vi "Begin.vi"(8 "error in":errorcluster) -> (0 "error out":errorcluster)   [LabVIEW 2019]
doc: "Called before other user functions, this VI is expected to open initial I/O refnums, load in file data, and do all program initialization. Notice that the <B>error out</B> terminal is simply used for data flow. Wiring it to other structures or subVIs ensures that this VI runs first."
uses:
  <vilib>/Rock Robotics/WPI/DriverStation/WPI_DriverStationRobotMode2.ctl
  <vilib>/Rock Robotics/WPI/Joystick/WPI_JoystickDeviceEnum.ctl
  <vilib>/Rock Robotics/SystemInterfaces/i2clib/i2c_bus.ctl
  <vilib>/Rock Robotics/WPI/ThirdParty/REV Robotics/Color SensorV3/Typedef/Color Sensor V3 LEDPulseFreq.ctl
  <vilib>/Rock Robotics/WPI/ThirdParty/REV Robotics/Color SensorV3/Typedef/Color Sensor V3 LEDCurrent.ctl
  <vilib>/Rock Robotics/SystemInterfaces/DIO/FPGA_DIOPWMChannel.ctl
  <vilib>/Rock Robotics/WPI/SafetyOutput/WPI_SafetyOutputConfigMenu.ctl
  <vilib>/Rock Robotics/SystemInterfaces/AI/FPGA_AIChannel.ctl
  <vilib>/Rock Robotics/WPI/Solenoid/WPI_SolenoidChannel.ctl
  Robot Global Data.vi
  <vilib>/Rock Robotics/Network Tables/NT Write String Array.vi
  Downloads/Global 2.vi
  <vilib>/Rock Robotics/WPI/Ultrasonic/WPI_SonarMB1010AnalogOpen.vi
  <vilib>/Rock Robotics/WPI/Ultrasonic/WPI_SonarMB1010AnalogRefNum Registry Set.vi
  <vilib>/Rock Robotics/WPI/MotorControl/WPI_MotorControlOpen VictorSPX.vi
  <vilib>/Rock Robotics/WPI/MotorControl/WPI_MotorControlOpen Talon.vi
  <vilib>/Rock Robotics/WPI/Solenoid/WPI_SolenoidOpenSingle.vi
  <vilib>/Rock Robotics/WPI/RobotDrive/WPI_RobotDriveOpen4MotorWithSPARK.vi
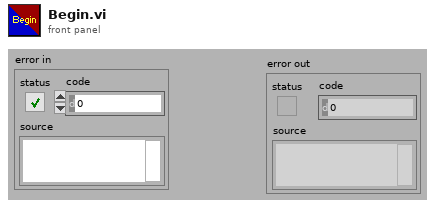
[diagram p1: front panel]
types:
  T1 = typedef "WPI_SolenoidChannel.ctl" = enum8{"Solenoid 0", "Solenoid 1", "Solenoid 2", "Solenoid 3", "Solenoid 4", "Solenoid 5", "Solenoid 6", "Solenoid 7", "Invalid"}
  T2 = typedef "FPGA_DIOPWMChannel.ctl" = enum8{"PWM 0", "PWM 1", "PWM 2", "PWM 3", "PWM 4", "PWM 5", "PWM 6", "PWM 7", "PWM 8", "PWM 9", "PWM MXP 0", "PWM MXP 1", "PWM MXP 2", "PWM MXP 3", "PWM MXP 4", "PWM MXP 5", "PWM MXP 6", "PWM MXP 7", "PWM MXP 8", "PWM MXP 9", "Invalid"}
  T3 = typedef "FPGA_AIChannel.ctl" = enum8{"AI 0", "AI 1", "AI 2", "AI 3", "AI MXP 0", "AI MXP 1", "AI MXP 2", "AI MXP 3", "Invalid"}
  T4 = typedef "WPI_SafetyOutputConfigMenu.ctl" = enum16{"Enable", "Disable"}
  T5 = typedef "Color Sensor V3 LEDCurrent.ctl" = enum8{"2.5mA", "5.0mA", "10mA", "25mA", "50mA", "75mA", "100mA", "125mA"}
  T6 = typedef "Color Sensor V3 LEDPulseFreq.ctl" = enum16{"60kHz", "70kHz", "80kHz", "90kHz", "100kHz"}
  T7 = typedef "i2c_bus.ctl" = enum16{"I2C On-Board", "I2C MXP", "Invalid"}
  T8 = typedef "WPI_JoystickDeviceEnum.ctl" = enum16{"USB 0", "USB 1", "USB 2", "USB 3", "USB 4", "USB 5"}
  T9 = typedef "WPI_DriverStationRobotMode2.ctl" = enum16{"Autonomous Disabled", "Autonomous Enabled", "Teleop Disabled", "Teleop Enabled", "Disconnected", "Finish", "Test Disabled", "Test Enabled", "Emergency Stopped"}
  T10 = typedef "WPI_RobotDriveDevRef.ctl" = cluster{"DevStatus":errorcluster, "Motors[]":T11[], "Square Inputs":bool, "Max Output":dbl}
  T11 = typedef "WPI_MotorControlDeviceRef.ctl" = cluster{"DeviceStatus":errorcluster, "Type":T12, "PWM":cluster{"PWM Channel":T2, "DeadBand":T13}, "CAN":cluster{"Device Number":u8, "SetOutput VI Ref":variant, "GetOutput VI Ref":variant, "Enable VI Ref":variant, "Disable VI Ref":variant, "Data":variant}, "Invert":bool, "DIO PWM":cluster{"PWM \"Enable\" Channel":T2, "DIOChannel":T14, "PWM Rate":dbl}}
  T12 = typedef "WPI_MotorControlType.ctl" = enum16{"PWM", "CAN", "DIO PWM"}
  T13 = typedef "WPI_PWMDeadband.ctl" = cluster{"Name":string, "maxPositivePwm":i32, "minPositivePwm":i32, "centerPwm":i32, "maxNegativePwm":i32, "minNegativePwm":i32, "angularRange":u16}
  T14 = typedef "FPGA_DIOChannel.ctl" = enum8{"DIO 0", "DIO 1", "DIO 2", "DIO 3", "DIO 4", "DIO 5", "DIO 6", "DIO 7", "DIO 8", "DIO 9", "DIO MXP 0", "DIO MXP 1", "DIO MXP 2", "DIO MXP 3", "DIO MXP 4", "DIO MXP 5", "DIO MXP 6", "DIO MXP 7", "DIO MXP 8", "DIO MXP 9", "DIO MXP 10", "DIO MXP 11", "DIO MXP 12", "DIO MXP 13", "DIO MXP 14", "DIO MXP 15", "SPI Port CS1", "SPI Port CS2", "SPI Port CS3", "SPI Port MISO", "SPI Port MOSI", "Invalid"}
  T15 = typedef "WPI_JoystickDevRef.ctl" = cluster{"Device":T8}
  T16 = typedef "Color Sensor V3 DevRef.ctl" = cluster{"I2CDevRef":T17}
  T17 = typedef "WPI_I2CDevRef.ctl" = cluster{"DevStatus":errorcluster, "Device Address":u8, "Handle":i32, "I2C Bus":T7}
  T18 = typedef "WPI_SolenoidDevRef.ctl" = cluster{"DevStatus":errorcluster, "Pneumatics Control Module":u8, "Forward Solenoid Channel":T1, "Reverse Solenoid Channel":T1}
  T19 = typedef "WPI_SonarMB1010AnalogDeviceRef.ctl" = cluster{"AIDeviceRef":T20, "Scaling factor (V/in)":dbl, "Average Bits":u8}
  T20 = typedef "WPI_AnalogChannelDevRef.ctl" = cluster{"DevStatus":errorcluster, "Analog Channel":T3}
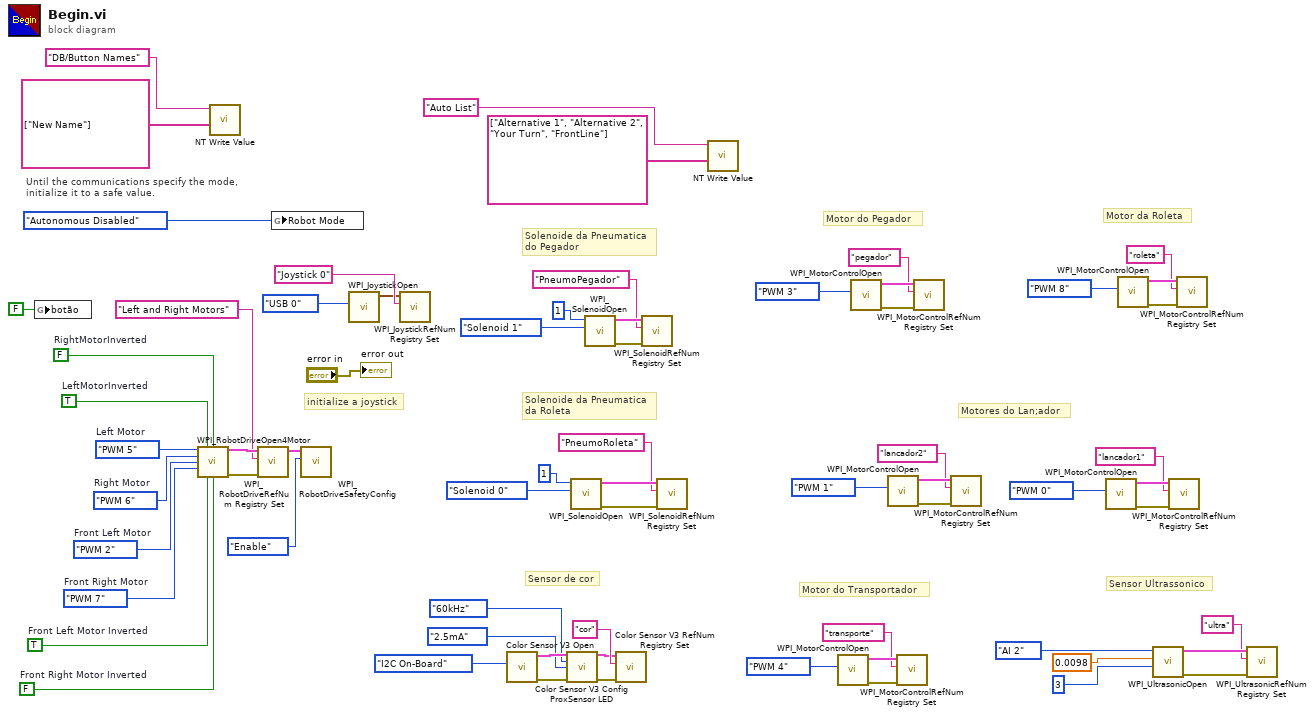
[diagram p0: block diagram]
diagram:
  w6 = FPGA_DIOPWMChannel."PWM 7"  # Front Right Motor
  w7 = FPGA_DIOPWMChannel."PWM 2"  # Front Left Motor
  w8 = FALSE  # Front Right Motor Inverted
  w9 = TRUE  # Front Left Motor Inverted
  w43 = FPGA_DIOPWMChannel."PWM 6"  # Right Motor
  w44 = FPGA_DIOPWMChannel."PWM 5"  # Left Motor
  w48 = TRUE  # LeftMotorInverted
  w49 = FALSE  # RightMotorInverted
  # "Sensor Ultrassonico"
  # "Motor do Transportador"
  # "Sensor de cor"
  # "Motores do Lan;ador"
  # "Motor da Roleta"
  # "Motor do Pegador"
  # "Solenoide da Pneumatica\nda Roleta"
  # "Solenoide da Pneumatica\ndo Pegador"
  # "initialize a joystick"
  # "Until the communications specify the mode,\ninitialize it to a safe value."
  n1 = global write "Global 2.vi" "botão"(FALSE ("botão")) -> ()
  n2 = call-poly <vilib>:"WPI_RobotDriveOpen4Motor.vi"("Rear Left Motor"=w44, "Rear Left Motor Inverted"=w48, "Rear Right Motor Inverted"=w49, "Rear Right Motor"=w43, "Front Left Motor"=w7, "Front Right Motor"=w6, "Front Left Motor Inverted"=w9, "Front Right Motor Inverted"=w8) -> ("RobotDriveDevRef"=w47:T10, "error out"=w45:errorcluster)  [unwired: 6 in]
  n3 = call-poly <vilib>:"NT Write Value.vi"("String Array"=string[] ["New Name"], "Name"="DB/Button Names") -> ()  [unwired: 9 in, 1 out]
  n4 = call <vilib>:"WPI_RobotDriveRefNum Registry Set.vi"("error in (no error)"=w45, "refnum name"="Left and Right Motors", "RobotDriveDevRef"=w47) -> ("RobotDriveDevRef"=w42:T10)  [unwired: 1 in, 7 out]
  n5 = global write "Robot Global Data.vi" "Robot Mode"(WPI_DriverStationRobotMode2."Autonomous Disabled" ("Robot Mode")) -> ()
  n6 = call <vilib>:"WPI_RobotDriveSafetyConfig.vi"("mode"=WPI_SafetyOutputConfigMenu."Enable", "RobotDriveDevRef"=w42) -> ()  [unwired: 8 in, 2 out]
  n7 = call <vilib>:"WPI_JoystickOpen.vi"("JoystickDevice"=WPI_JoystickDeviceEnum."USB 0") -> ("JoystickDevRef"=w65:T15)  [unwired: 10 in]
  n8 = call <vilib>:"WPI_JoystickRefNum Registry Set.vi"("refnum name"="Joystick 0", "JoystickDevRef"=w65) -> ()  [unwired: 8 in, 2 out]
  n9 = call <vilib>:"Color Sensor V3 Open.vi"("I2C Bus"=i2c_bus."I2C On-Board") -> ("error out"=w54:errorcluster, "ColorSensorDevRef"=w53:T16)  [unwired: 9 in]
  n10 = call <vilib>:"Color Sensor V3 Config ProxSensor LED.vi"("ColorSensorDevRef"=w53, "LEDPulseFreq"=Color_Sensor_V3_LEDPulseFreq."60kHz", "LEDCurrent"=Color_Sensor_V3_LEDCurrent."2.5mA", "error in (no error)"=w54) -> ("ColorSensorDevRef out"=w56:T16, "error out"=w55:errorcluster)  [unwired: 10 in]
  n11 = call-poly <vilib>:"WPI_SolenoidOpen.vi"("Solenoid Channel"=WPI_SolenoidChannel."Solenoid 0", "Pneumatics Control Module (0)"=u8 1) -> ("error out"=w18:errorcluster, "SolenoidDevRef"=w17:T18)  [unwired: 8 in]
  n12 = call-poly <vilib>:"WPI_SolenoidOpen.vi"("Solenoid Channel"=WPI_SolenoidChannel."Solenoid 1", "Pneumatics Control Module (0)"=u8 1) -> ("error out"=w5:errorcluster, "SolenoidDevRef"=w4:T18)  [unwired: 8 in]
  n13 = call <vilib>:"Color Sensor V3 RefNum Registry Set.vi"("error in (no error)"=w55, "refnum name"="cor", "ColorSensorDevRef"=w56) -> ()  [unwired: 7 in, 2 out]
  n14 = call <vilib>:"WPI_SolenoidRefNum Registry Set.vi"("error in (no error)"=w5, "refnum name"="PneumoPegador", "SolenoidDevRef"=w4) -> ()  [unwired: 7 in, 2 out]
  n15 = call <vilib>:"WPI_SolenoidRefNum Registry Set.vi"("error in (no error)"=w18, "refnum name"="PneumoRoleta", "SolenoidDevRef"=w17) -> ()  [unwired: 7 in, 2 out]
  n16 = call-poly <vilib>:"NT Write Value.vi"("String Array"=string[] ["Alternative 1", "Alternative 2", "Your Turn", "FrontLine"], "Name"="Auto List") -> ()  [unwired: 9 in, 1 out]
  n17 = call-poly <vilib>:"WPI_MotorControlOpen.vi"("PWM Channel"=FPGA_DIOPWMChannel."PWM 4") -> ("error out"=w13:errorcluster, "MotorControlDeviceRef"=w12:T11)  [unwired: 9 in]
  n18 = call-poly <vilib>:"WPI_MotorControlOpen.vi"("PWM Channel"=FPGA_DIOPWMChannel."PWM 3") -> ("error out"=w34:errorcluster, "MotorControlDeviceRef"=w33:T11)  [unwired: 9 in]
  n19 = call-poly <vilib>:"WPI_MotorControlOpen.vi"("PWM Channel"=FPGA_DIOPWMChannel."PWM 1") -> ("error out"=w22:errorcluster, "MotorControlDeviceRef"=w21:T11)  [unwired: 9 in]
  n20 = call <vilib>:"WPI_MotorControlRefNum Registry Set.vi"("error in (no error)"=w13, "refnum name"="transporte", "MotorControlDevRef"=w12) -> ()  [unwired: 7 in, 2 out]
  n21 = call <vilib>:"WPI_MotorControlRefNum Registry Set.vi"("error in (no error)"=w34, "refnum name"="pegador", "MotorControlDevRef"=w33) -> ()  [unwired: 7 in, 2 out]
  n22 = call <vilib>:"WPI_MotorControlRefNum Registry Set.vi"("error in (no error)"=w22, "refnum name"="lancador2", "MotorControlDevRef"=w21) -> ()  [unwired: 7 in, 2 out]
  n23 = call-poly <vilib>:"WPI_MotorControlOpen.vi"("PWM Channel"=FPGA_DIOPWMChannel."PWM 0") -> ("error out"=w26:errorcluster, "MotorControlDeviceRef"=w25:T11)  [unwired: 9 in]
  n24 = call-poly <vilib>:"WPI_MotorControlOpen.vi"("PWM Channel"=FPGA_DIOPWMChannel."PWM 8") -> ("error out"=w30:errorcluster, "MotorControlDeviceRef"=w29:T11)  [unwired: 9 in]
  n25 = call-poly <vilib>:"WPI_UltrasonicOpen.vi"("Average Bits"=u8 3, "Scaling factor (V/in)"=0.0098, "Analog Channel"=FPGA_AIChannel."AI 2") -> ("error out"=w40:errorcluster, "SonarMB1010AnalogDevRef"=w39:T19)  [unwired: 7 in]
  n26 = call <vilib>:"WPI_MotorControlRefNum Registry Set.vi"("error in (no error)"=w26, "refnum name"="lancador1", "MotorControlDevRef"=w25) -> ()  [unwired: 7 in, 2 out]
  n27 = call <vilib>:"WPI_MotorControlRefNum Registry Set.vi"("error in (no error)"=w30, "refnum name"="roleta", "MotorControlDevRef"=w29) -> ()  [unwired: 7 in, 2 out]
  n28 = call-poly <vilib>:"WPI_UltrasonicRefNum Registry Set.vi"("error in (no error)"=w40, "refnum name"="ultra", "SonarMB1010AnalogDevRef"=w39) -> ()  [unwired: 7 in, 2 out]
  "error out" <- "error in"
